vi "Imgaussfilt.vi"(9 "sigma":dbl, 11 "X":dbl[][](array[numeric])) -> (3 "Y":dbl[][](array[numeric]))   [LabVIEW 2020]
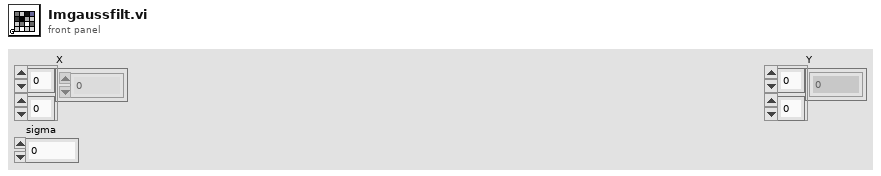
[diagram p1: front panel]
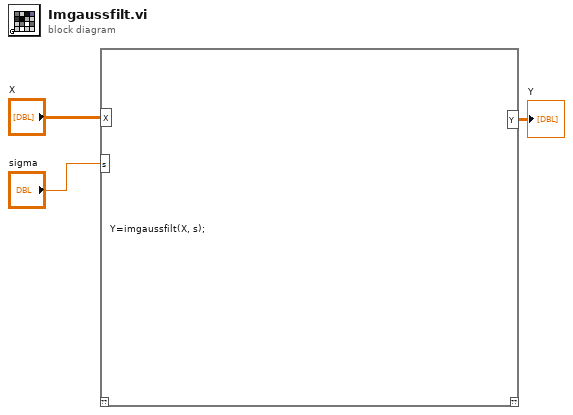
[diagram p0: block diagram]
diagram:
  n1 = script code="Y=imgaussfilt(X, s);"("X"="X", "s"="sigma") -> ("Y"=→"Y":dbl[][])  [unwired: 1 in, 1 out]
